vi "2_KIT_covid_19_modificado_para_subpanel.vi"() -> ()   [LabVIEW 2019]
panel:
  out "Array_INI":bool[](array[boolean])
  in  "stop":bool
  out "Array_OUT":bool[](array[boolean])
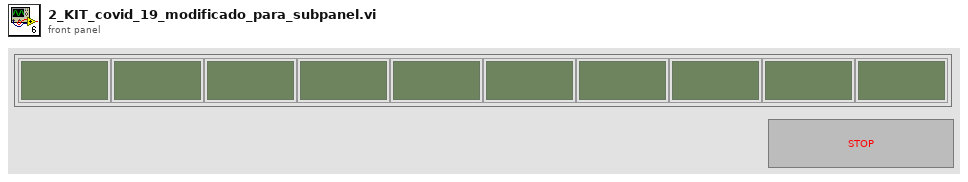
[diagram p1: front panel]
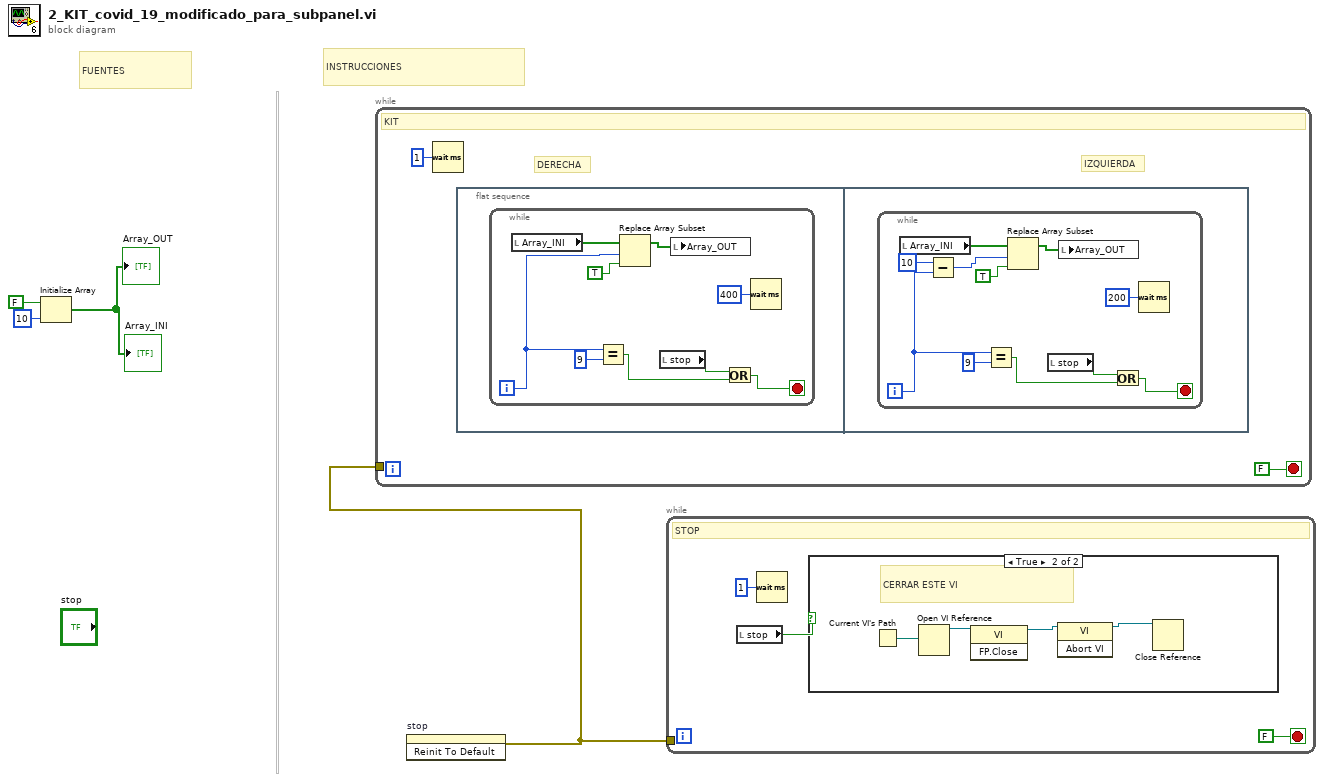
[diagram p0: block diagram]
diagram:
  # "INSTRUCCIONES"
  # "FUENTES"
  n1 = Initialize Array(FALSE, 10 ("dimension size")) -> (→"Array_OUT" →"Array_INI":bool[])
  n2 = invoke on="stop" class="Bool (strict)" method="Reinit To Default"() -> (error out=w4:errorcluster)  [unwired: 3 in, 2 out]
  n3 = while {
    tunnel: w4 -> [_]
    stop <- FALSE stop-if-true
    # "IZQUIERDA"
    # "DERECHA"
    # "KIT"
    n4 = Wait (ms)(milliseconds to wait=u32 1) -> ()  [unwired: 1 out]
    n5 = flat-sequence {
      frame #0 {
        n6 = while {
          i -> [w11]
          stop <- w9 stop-if-true
          n7 = local read "Array_INI"() -> (w15:bool[])
          n8 = Equal?(x=w11, y=9) -> (x = y?=w8:bool)
          n9 = Replace Array Subset(array=w15, new element=TRUE, index=w11) -> (w14:bool[])
          n10 = local read "stop"() -> (w7:bool)
          n11 = local write "Array_OUT"(w14) -> ()
          n12 = Or(x=w7, y=w8) -> (x .or. y?=w9:bool)
          n13 = Wait (ms)(milliseconds to wait=u32 400) -> ()  [unwired: 1 out]
        }
      }
      frame #1 {
        n14 = while {
          i -> [w18]
          stop <- w21 stop-if-true
          n15 = local read "Array_INI"() -> (w26:bool[])
          n16 = Subtract(x=10, y=w18) -> (x-y=w16:i32)
          n17 = Equal?(x=w18, y=9) -> (x = y?=w20:bool)
          n18 = Replace Array Subset(array=w26, new element=TRUE, index=w16) -> (w25:bool[])
          n19 = local read "stop"() -> (w19:bool)
          n20 = local write "Array_OUT"(w25) -> ()
          n21 = Or(x=w19, y=w20) -> (x .or. y?=w21:bool)
          n22 = Wait (ms)(milliseconds to wait=u32 200) -> ()  [unwired: 1 out]
        }
      }
    }
  }
  n23 = while {
    tunnel: w4 -> [_]
    stop <- FALSE stop-if-true
    # "STOP"
    n24 = local read "stop"() -> (w28:bool)
    n25 = Wait (ms)(milliseconds to wait=u32 1) -> ()  [unwired: 1 out]
    n26 = case shown="True" w28 {
      frame False {
      }
      frame True {
        # "CERRAR ESTE VI"
        n27 = Current VI's Path() -> (path=w33:path)
        n28 = Open VI Reference(vi path=w33) -> (vi reference=w31:refnum<vi>)  [unwired: 5 in, 1 out]
        n29 = invoke class="VI" method="FP.Close"(reference=w31) -> (reference out=w30:refnum<vi>)  [unwired: 2 in, 2 out]
        n30 = invoke class="VI" method="Abort VI"(reference=w30) -> (reference out=w32:refnum<vi>)  [unwired: 2 in, 2 out]
        n31 = Close Reference(reference=w32) -> ()  [unwired: 1 in, 1 out]
      }
    }
  }
